vi "Merge Data.vi"(8 "error in":errorcluster, 10 "Analyzed":refnum<class "Instrument.lvclass">, 11 "Acquired":refnum<class "Aircraft OPCCRD.lvclass">) -> (0 "error out":errorcluster, 3 "tCRD out":refnum<class "Aircraft OPCCRD.lvclass">)   [LabVIEW 2015, in "Aircraft OPCCRD.lvclass"]
doc: "The VI Merge Data is used strictly here to merge the serial data with the rest of the data. THIS VI WILL BE NO LONGER NECESSARY WHEN ISSUES RELATING TO RT EXE ARE FIXED!!"
uses:
  Aircraft OPCCRD.lvclass
  Reusable/Instrument/Instrument.lvclass
  Aircraft OPCCRD.lvclass/Aircraft OPCCRD.ctl
  Reusable/CRDS/Main/CRDS.lvclass
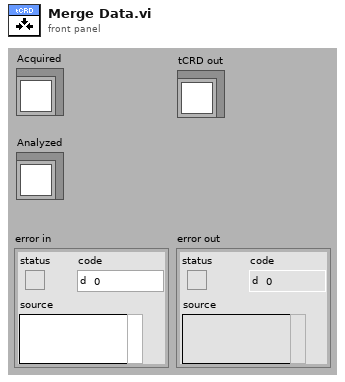
[diagram p1: front panel]
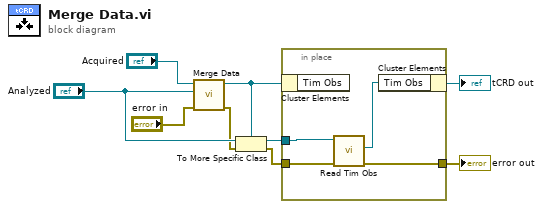
[diagram p0: block diagram]
diagram:
  n1 = call-parent "Merge Data.vi"("error in"="error in", "Analyzed"="Analyzed", "Acquired"="Acquired") -> ("error out"=w4:errorcluster, "CRDS out"=w1:refnum<class "Aircraft OPCCRD.lvclass">)  [unwired: 7 in]
  n2 = To More Specific Class(target class=w1, reference="Analyzed", error in=w4) -> (specific class reference=w6:refnum<class "Aircraft OPCCRD.lvclass">, error out=w3:errorcluster)
  n3 = in-place {
    in-place-border: w6 -> [w13]
    in-place-border: w3 -> [w11]
    in-place-border: [w10] -> w2
    n4 = in-place-cluster #1(w1) -> ()  [unwired: 1 out]
    n5 = call "Read Tim Obs.vi"("error in"=w11, "tCRD in"=w13) -> ("error out"=w10:errorcluster, "Tim Obs"=w12:refnum<class "Tim File Observer.lvclass">)  [unwired: 7 in, 1 out]
    n6 = in-place-cluster #1("Tim Obs"=w12) -> (→"tCRD out":refnum<class "Aircraft OPCCRD.lvclass">)
  }
  "error out" <- w2
